vi "UnitTest-LogicSizeAsRoot.vi"(8 "error in (no error)":errorcluster, 10 "LV Data":T1, 11 ">> Config >>":T2={"TableLogger"=enum."SQLite Logger", "DB File Path"=path "DB.db", "DB Backup Config"={"Directory"=path "DB/Backup", "UTC Time Format"=FALSE, "On Launch"=FALSE, "Interval (Hours)"=-1.0, "Size Multiples (Bytes)"=10000}}) -> (0 "error out":errorcluster, 2 "Dir?T":bool, 3 "DataSize?Equal":bool)   [LabVIEW 2014]
uses:
  TableLogger_Actor/TableLoggerConfig.ctl
  TableLogger_Actor/TableLoggerTypes.ctl
  TableLogger_Actor/TableLoggerBackupConfig.ctl
  TableLogger_Actor/TableLoggerDataCluster.ctl
  <vilib>/ActorFramework/Message Enqueuer/Message Enqueuer.lvclass/Message Enqueuer.ctl
  <vilib>/ActorFramework/Message Enqueuer/Enqueue.vi
  <vilib>/ActorFramework/Message Priority Queue/Priority Enqueue.vi
  <vilib>/ActorFramework/Stop Msg/Stop Msg.lvclass
  TableLogger_Actor/TableLogger_Actor/TableLogger_Actor.lvclass
  TableLogger_Actor/TableLogger_Actor.lvlib
panel:
  # "Connector Pane"
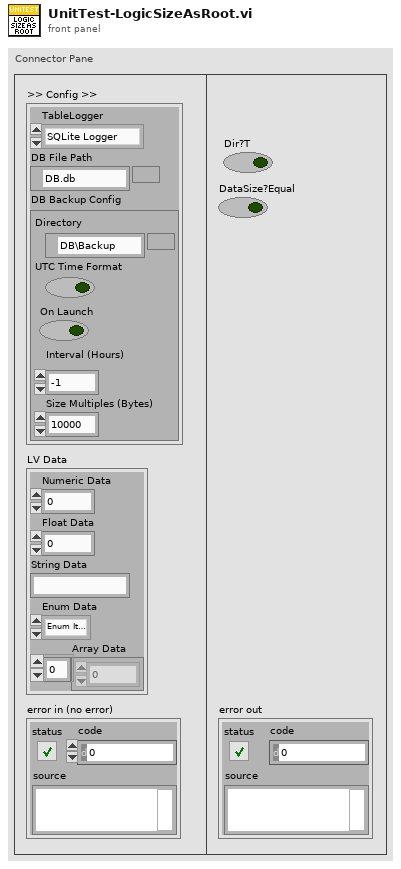
[diagram p1: front panel]
types:
  T1 = typedef "TableLogger_Actor.lvlib/TableLoggerDataCluster.ctl" = cluster{"Numeric Data":i32, "Float Data":dbl, "String Data":string, "Enum Data":enum16{"Enum Item 1", "Enum Item 2"}, "Array Data":i32[]}
  T2 = typedef "TableLogger_Actor.lvlib/TableLoggerConfig.ctl" = cluster{"TableLogger":T3, "DB File Path":path, "DB Backup Config":T4}
  T3 = typedef "TableLogger_Actor.lvlib/TableLoggerTypes.ctl" = enum16{"CSV Logger", "SQLite Logger"}
  T4 = typedef "TableLogger_Actor.lvlib/TableLoggerBackupConfig.ctl" = cluster{"Directory":path, "UTC Time Format":bool, "On Launch":bool, "Interval (Hours)":dbl, "Size Multiples (Bytes)":i32}
  T5 = typedef "File Info Record__ogtk.ctl" = cluster{"type":string, "creator":string, "permissions":i32, "data size":i32, "res size":i32, "creation date":u32, "modification date":u32, "bFolder":bool, "bInvisible":bool, "location":cluster{"vertical":i16, "horizontal":i16}, "owner":string, "group":string}
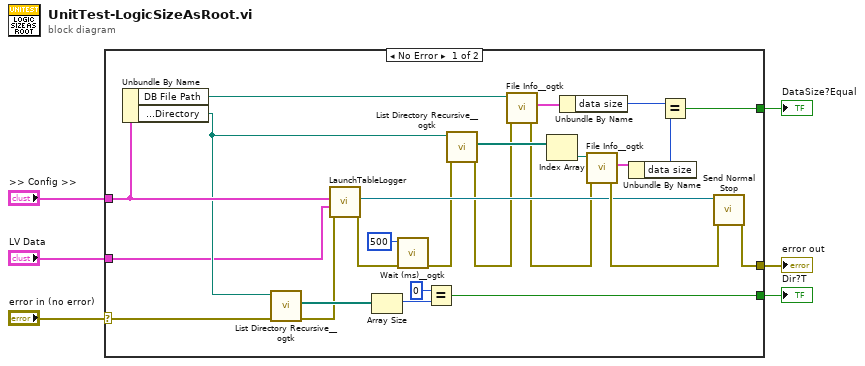
[diagram p0: block diagram]
diagram:
  n1 = case shown="No Error" "error in (no error)" {
    selector: "error in (no error)" -> [w25 _]
    tunnel: ">> Config >>" -> [w30 _]
    tunnel: [w27 _] -> w5
    tunnel: [w18 _] -> w3
    tunnel: [w15 _] -> w2
    tunnel: "LV Data" -> [w7 _]
    frame No Error {
      n2 = Unbundle By Name(w30) -> ("DB File Path"=w28:path, "DB Backup Config.Directory"=w29:path)
      n3 = call <userlib>:"List Directory Recursive__ogtk.vi"("error in (no error)"=w25, "Path"=w29) -> ("error out"=w11:errorcluster, "file paths"=w12:path[])  [unwired: 6 in, 2 out]
      n4 = call "LaunchTableLogger.vi"("error in (no error)"=w11, "Data Cluster (for Headers)"=w7, "TableLogger Config"=w30) -> ("error out"=w14:errorcluster, "TableLogger Actor's Enqueuer"=w26:refnum<class "Message Enqueuer.lvclass">)  [unwired: 5 in, 2 out]
      n5 = Array Size(array=w12) -> (size(s)=w24:i32)
      n6 = call <userlib>:"Wait (ms)__ogtk.vi"("error in (no error)"=w14, "milliseconds to wait"=u32 500) -> ("error out"=w13:errorcluster)  [unwired: 8 in, 1 out]
      n7 = Equal?(x=0, y=w24) -> (x = y?=w18:bool)
      n8 = call <userlib>:"List Directory Recursive__ogtk.vi"("error in (no error)"=w13, "Path"=w29) -> ("error out"=w9:errorcluster, "file paths"=w22:path[])  [unwired: 6 in, 2 out]
      n9 = call <userlib>:"File Info__ogtk.vi"("error in (no error)"=w9, "file"=w28) -> ("error out"=w8:errorcluster, "file info"=w19:T5)  [unwired: 4 in, 1 out]
      n10 = Index Array(array=w22) -> (element=w21:path)  [unwired: 1 in]
      n11 = Unbundle By Name(w19) -> ("data size"=w17:i32)
      n12 = call <userlib>:"File Info__ogtk.vi"("error in (no error)"=w8, "file"=w21) -> ("error out"=w31:errorcluster, "file info"=w20:T5)  [unwired: 4 in, 1 out]
      n13 = Unbundle By Name(w20) -> ("data size"=w16:i32)
      n14 = Equal?(x=w17, y=w16) -> (x = y?=w15:bool)
      n15 = call <vilib>:"Send Normal Stop.vi"("error in (no error)"=w31, "Message Enqueuer"=w26) -> ("error out"=w27:errorcluster)  [unwired: 9 in]
    }
    frame Error {
    }
  }
  "error out" <- w5
  "Dir?T" <- w3
  "DataSize?Equal" <- w2
